vi "No_linealidades.vi"() -> ()   [LabVIEW 2013]
uses:
  <vilib>/platform/TimedLoop/XDataNode/XDataNode.xnode
  <vilib>/Platform/TimedLoop/XDataNode/nitl_modes.ctl
  <vilib>/Platform/TimedLoop/XDataNode/XDNodeRunTimeDep.lvlib
  <vilib>/Platform/TimedLoop/XDataNode/wakeup.ctl
  <vilib>/Platform/TimedLoop/XDataNode/timing_clust.ctl
  <vilib>/DAQmx/create/channels.llb/DAQmx Create Channel (DO-Digital Output).vi
  <vilib>/DAQmx/write.llb/DAQmx Write (Digital Bool 1Line 1Point).vi
  <vilib>/DAQmx/read.llb/DAQmx Read (Counter DBL 1Chan 1Samp).vi
  <vilib>/DAQmx/create/channels.llb/DAQmx Create Channel (CI-Position-Angular Encoder).vi
  <vilib>/DAQmx/configure/timing.llb/DAQmx Timing (Implicit).vi
  <vilib>/DAQmx/create/channels.llb/DAQmx Create Channel (CO-Pulse Generation-Frequency).vi
  <vilib>/DAQmx/write.llb/DAQmx Write (Counter Frequency 1Chan 1Samp).vi
panel:
  in  "counter":tag
  in  "lines":tag
  out "Valor duty cycle":dbl[](array[numeric])
  out "Finished Late? [i-1]":bool
  out "Iteration Duration":i64
  out "Numeric":i32
  in  "Stop":bool
  out "Tick por Tm":dbl
  in  "auto start 2":bool=TRUE
  in  "auto start":bool=TRUE
  in  "pulses per revolution":u32=24
  in  "Numero de muestras de PWM":dbl
  out "Waveform Graph 2":waveform(dbl)(graph)
  in  "physical channels":tag
  in  "units":i32(ring)=10348 items=["Volts"=10348, "From Custom Scale"=10065]
  in  "Duración de los ceros":dbl=5.0
  in  "Duración de ciclo (s)":dbl=20.0
  in  "Periodo de muestreo":dbl=0.05
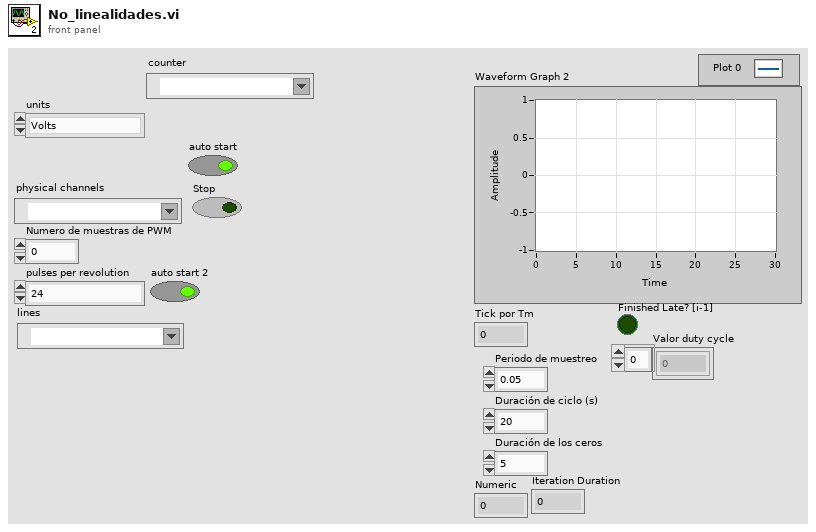
[diagram p1: front panel]
types:
  T1 = typedef "XDNodeRunTimeDep.lvlib/timing_clust.ctl" = cluster{"Expected End [f-1]":u64, "Actual End [f-1]":u64, "Finished Late? [f-1]":bool, "Expected End [i-1]":u64, "Actual End [i-1]":u64, "Finished Late? [i-1]":bool, "Expected Start [i]":u64, "Actual Start [i]":u64, "Expected Start [f]":u64, "Actual Start [f]":u64, "Source Name":string, "Structure Name":string, "Period":i64, "Deadline":i64, "Offset":i64, "Start":i64, "Priority":i32, "Timeout":i32, "Mode":T2, "Wakeup Reason":T3, "Error":errorcluster, "Source Type":string, "Secondary Source Type":string, "Global End Time":u64, "Global Start Time":u64, "Frame Duration":u64, "Iteration Duration":u64, "Assigned CPU":i32, "I/O Scan Engine Mode":u32}
  T2 = typedef "XDNodeRunTimeDep.lvlib/nitl_modes.ctl" = enum32{"No Change", "Process missed periods, maintain original phase", "Discard missed periods, maintain original phase", "Process missed periods, ignore original phase", "Discard missed periods, ignore original phase"}
  T3 = typedef "XDNodeRunTimeDep.lvlib/wakeup.ctl" = enum32{"Normal", "Aborted", "Asynchronous wakeup", "Timing source error", "Timed loop error", "Timeout"}
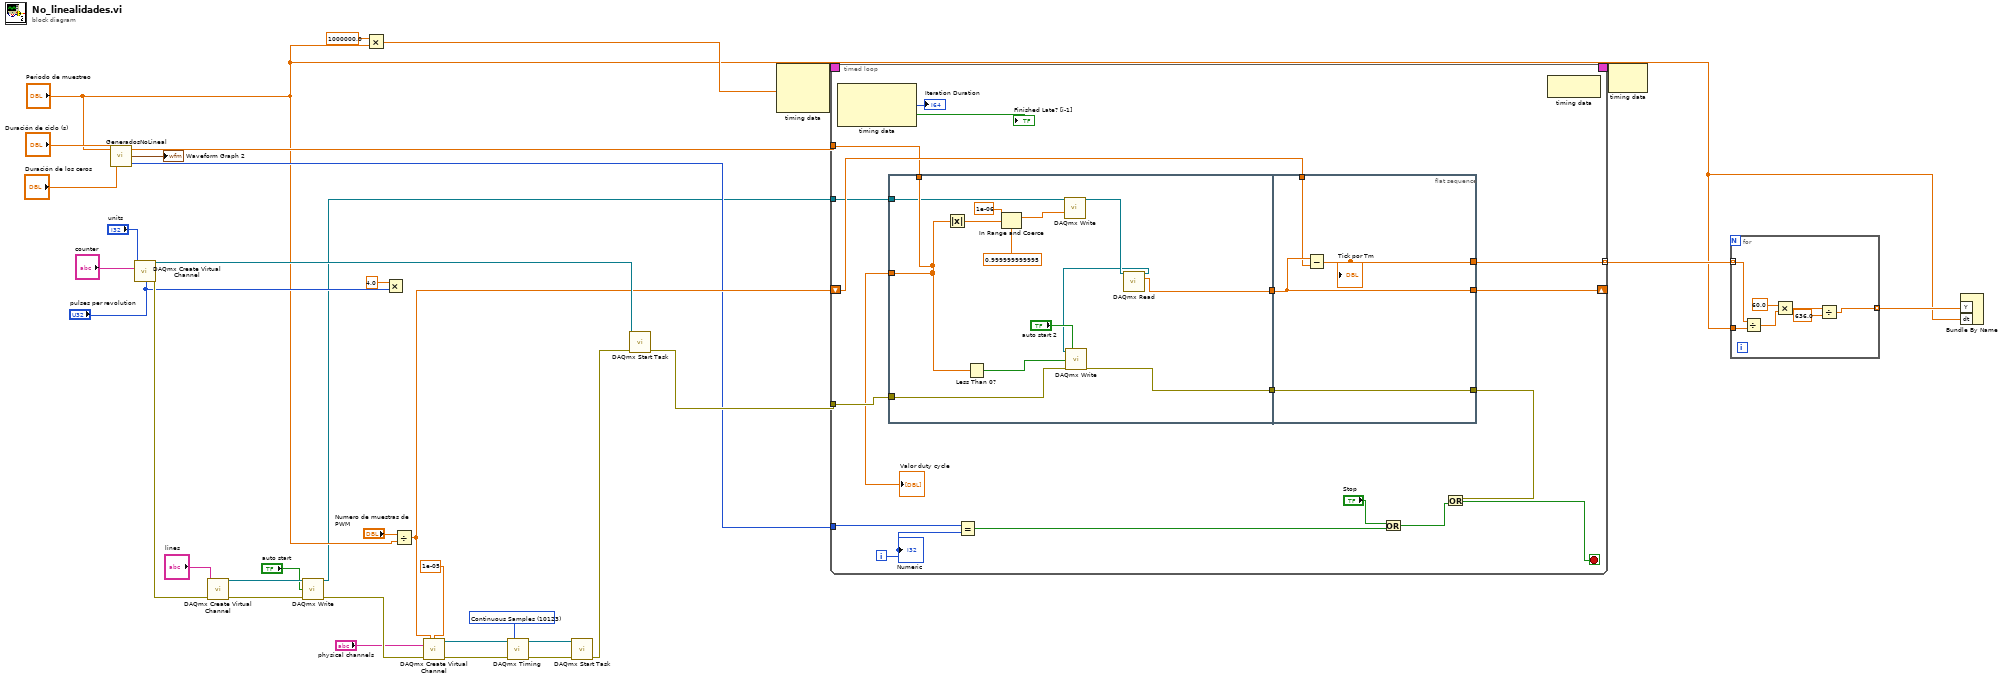
[diagram p0: block diagram]
diagram:
  w18 = 10123 items=["Finite Samples"=10178, "Continuous Samples"=10123, "Hardware Timed Single Point"=12522] ("sample mode")
  n1 = call "GeneradosNoLineal.vi"("Duración de los ceros"="Duración de los ceros", "Duración de ciclo (s)"="Duración de ciclo (s)", "Periodo de muestreo"="Periodo de muestreo") -> ("Numero de muestras"=w7:i32, "Waveform Graph 2"=→"Waveform Graph 2":waveform(dbl), "Señal No linealidad"=w8:dbl[])
  n2 = call-poly <vilib>:"DAQmx Create Virtual Channel.vi"("counter"="counter", "units"="units", "pulses per revolution"="pulses per revolution") -> ("task out"=w21:refnum<k21>, "error out"=w30:errorcluster)  [unwired: 11 in]
  n3 = call-poly <vilib>:"DAQmx Create Virtual Channel.vi"("lines"="lines", "error in"=w30) -> ("task out"=w28:refnum<k21>, "error out"=w29:errorcluster)  [unwired: 12 in]
  n4 = call-poly <vilib>:"DAQmx Write.vi"("task/channels in"=w28, "data"="auto start", "error in"=w29) -> ("task out"=w4:refnum<k21>, "error out"=w27:errorcluster)  [unwired: 10 in, 1 out]
  n5 = Multiply(x=1000000.0, y="Periodo de muestreo") -> (x*y=w13:dbl)
  n6 = Multiply(x=4.0, y="pulses per revolution") -> ()  [unwired: 1 out]
  n7 = Divide(x="Numero de muestras de PWM", y="Periodo de muestreo") -> (x/y=w9:dbl)
  n8 = call-poly <vilib>:"DAQmx Create Virtual Channel.vi"("frequency"=w9, "duty cycle"=1e-05 ("frequency"), "counter"="physical channels", "error in"=w27) -> ("task out"=w24:refnum<k21>, "error out"=w25:errorcluster)  [unwired: 10 in]
  n9 = call-poly <vilib>:"DAQmx Timing.vi"("task/channels in"=w24, "sample mode"=w18, "error in"=w25) -> ("task out"=w22:refnum<k21>, "error out"=w23:errorcluster)  [unwired: 11 in]
  n10 = call <vilib>:"DAQmx Start Task.vi"("task/channels in"=w22, "error in"=w23) -> ("error out"=w20:errorcluster)  [unwired: 12 in, 1 out]
  n11 = call <vilib>:"DAQmx Start Task.vi"("task/channels in"=w21, "error in"=w20) -> ("error out"=w10:errorcluster)  [unwired: 12 in, 1 out]
  n12 = node-c288(w13) -> (w35:T1)  [unwired: 2 in]
  n13 = timed-loop {
    timing: w35 -> [_]
    timing-out: [_] -> w34
    shift-right: [w51] -> _
    shift-left: w9 -> [w46]
    tunnel: [w52] -> w11 mode=indexing
    tunnel: w10 -> [w43]
    tunnel: w8 -> [w39]
    tunnel: w7 -> [w37]
    tunnel: w4 -> [w36]
    i -> [w42]
    stop <- w50 stop-if-true
    n14 = node-c288() -> (→"Iteration Duration":i64, →"Finished Late? [i-1]":bool)  [unwired: 1 in, 1 out]
    n15 = flat-sequence {
      tunnel: [w61] -> w53
      tunnel: [w58] -> w38
      tunnel: [w59] -> w44
      tunnel: w43 -> [w60]
      tunnel: w39 -> [w58]
      tunnel: w36 -> [w54]
      tunnel: w53 -> [w69]
      tunnel: [w70] -> w52
      tunnel: [w69] -> w51
      tunnel: w46 -> [w68]
      tunnel: [w67] -> w45
      tunnel: w44 -> [w67]
      frame #0 {
        n16 = Absolute Value(x=w58) -> (abs(x)=w66:dbl[])
        n17 = Less Than 0?(x=w58) -> (x < 0?=w57:bool[])
        n18 = In Range and Coerce(upper limit=1e-06, x=w66, lower limit=0.999999999995) -> (coerced(x)=w65:dbl[])  [unwired: 1 out]
        n19 = call-poly <vilib>:"DAQmx Write.vi"("task/channels in"=w54, "timeout"=w65) -> ("task out"=w56:refnum<k21>)  [unwired: 11 in, 2 out]
        n20 = call-poly <vilib>:"DAQmx Read.vi"("task/channels in"=w56) -> ("task out"=w55:refnum<k21>, "data"=w61:dbl)  [unwired: 12 in, 1 out]
        n21 = call-poly <vilib>:"DAQmx Write.vi"("task/channels in"=w55, "auto start"="auto start 2", "data"=w57, "error in"=w60) -> ("error out"=w59:errorcluster)  [unwired: 9 in, 2 out]
      }
      frame #1 {
        n22 = Subtract(x=w69, y=w68) -> (x-y=w70:dbl)
        "Tick por Tm" <- w70
      }
    }
    n23 = Equal?(x=w37, y=w42) -> (x = y?=w48:bool)
    n24 = Or(x="Stop", y=w48) -> (x .or. y?=w49:bool)
    n25 = Or(x=w45, y=w49) -> (x .or. y?=w50:bool)
    n26 = node-c288() -> ()  [unwired: 1 in, 1 out]
    "Numeric" <- w42
    "Valor duty cycle" <- w38
  }
  n27 = node-c288(w34) -> ()  [unwired: 1 out]
  n28 = for {
    tunnel: w11 -> [w77] mode=indexing
    tunnel: [w76] -> w6 mode=indexing
    tunnel: "Periodo de muestreo" -> [w75]
    n29 = Divide(x=w77, y=w75) -> (x/y=w81:dbl)
    n30 = Multiply(x=60.0, y=w81) -> (x*y=w79:dbl)
    n31 = Divide(x=w79, y=636.0) -> (x/y=w76:dbl)
  }
  n32 = Bundle By Name("Y"=w6, "dt"="Periodo de muestreo") -> ()  [unwired: 1 in, 1 out]
